vi "Mask LP filter.vi"() -> ()   [LabVIEW 2016]
uses:
  <vilib>/Analysis/2dsp.llb/2D Convolution (DBL).vi
  <vilib>/Analysis/NI_AALPro.lvlib
panel:
  in  "Xdim":dbl=10.0
  in  "Ydim":dbl=50.0
  in  "Val":dbl=0.002
  out "size(s)":i32[](array[numeric])=[180, 1000]
  out "Mask  2":dbl[][](graph)
  in  "Mask":dbl[][](graph)=array180x1000[180000 elements]
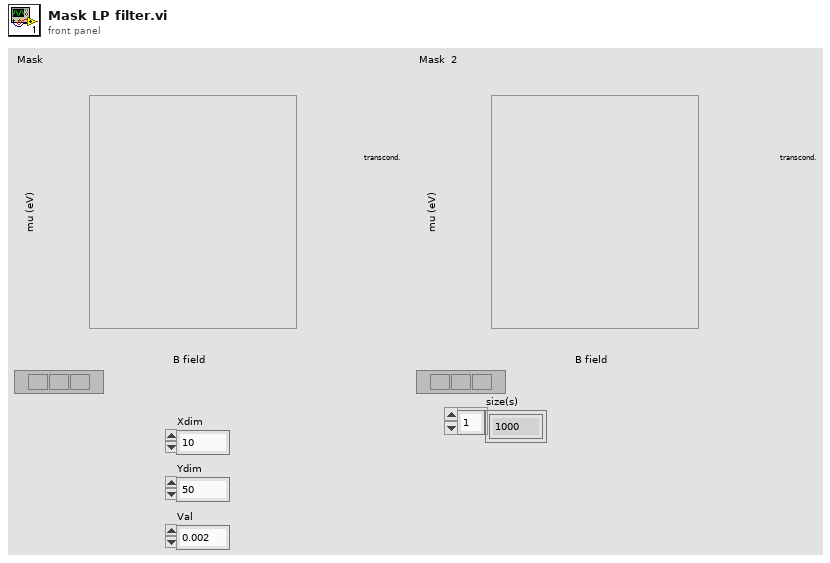
[diagram p1: front panel]
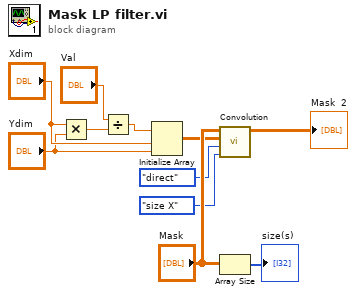
[diagram p0: block diagram]
diagram:
  n1 = Multiply(x="Xdim", y="Ydim") -> (x*y=w3:dbl)
  n2 = Divide(x="Val", y=w3) -> (x/y=w1:dbl)
  n3 = Initialize Array(w1, "Xdim", "Ydim") -> (w6:dbl[][])
  n4 = call-poly <vilib>:"Convolution.vi"("output size"=enum32{"full", "size X", "compact"}."size X", "algorithm"=enum32{"direct", "frequency domain"}."direct", "Y"=w6, "X"="Mask") -> ("X * Y"=→"Mask  2":dbl[][])  [unwired: 6 in, 1 out]
  n5 = Array Size(array="Mask") -> (size(s)=→"size(s)":i32[])
